vi "randn-vector.vi"(1 "Numeric":i32) -> (0 "Array":dbl[](array[numeric]))   [LabVIEW 2023]
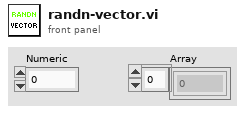
[diagram p1: front panel]
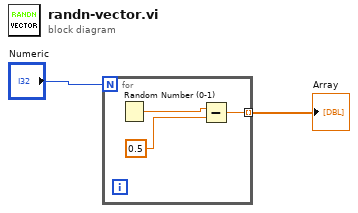
[diagram p0: block diagram]
diagram:
  n1 = for {
    N: "Numeric" -> [_]
    tunnel: [w3] -> w1 mode=indexing
    n2 = Random Number (0-1)() -> (number: 0 to 1=w4:dbl)
    n3 = Subtract(x=w4, y=0.5) -> (x-y=w3:dbl)
  }
  "Array" <- w1
